vi "libssh2_session_hostkey.vi"(8 "error in (no error)":errorcluster, 11 "session":T1) -> (0 "error out":errorcluster, 1 "type":i32, 2 "hostkey":u8[](array[numeric]))   [LabVIEW 2017, in "libssh2.lvlib"]
doc: "Get the host key of the remote host.\n\nUse this output with libssh2_knownhost_checkp and continue only when the known host check result is MATCH."
uses:
  libssh2.lvlib
  Session Refnum.ctl
  Not A Session.vi
  <vilib>/Utility/error.llb/Error Cluster From Error Code.vi
  Global Settings.vi
  Read Session Refnum.vi
  <vilib>/Utility/semaphor.llb/Acquire Semaphore.vi
  <vilib>/Utility/semaphor.llb/Release Semaphore.vi
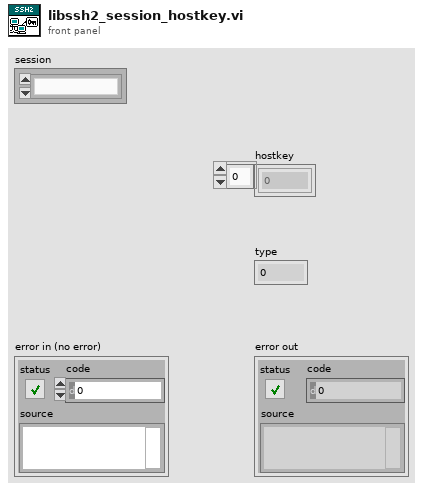
[diagram p1: front panel]
types:
  T1 = typedef "libssh2.lvlib/Session Refnum.ctl" = refnum<k1>
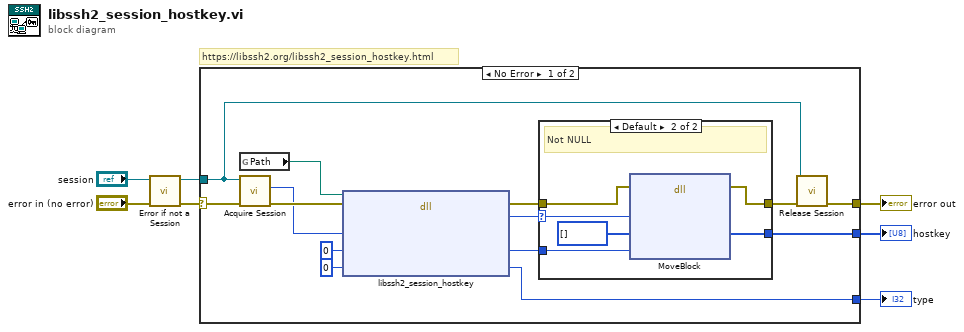
[diagram p0: block diagram]
diagram:
  # "https://libssh2.org/libssh2_session_hostkey.html"
  n1 = call "Error if not a Session.vi"("error in (no error)"="error in (no error)", "session"="session") -> ("error out"=w3:errorcluster, "session out"=w1:T1)  [unwired: 8 in]
  n2 = case shown="No Error" w3 {
    selector: w3 -> [w18 w29]
    tunnel: [w21 _] -> w7
    tunnel: [w9 w29] -> w6
    tunnel: [w19 _] -> w5
    tunnel: w1 -> [w8 _]
    frame No Error {
      n3 = global read "Global Settings.vi" "Path"() -> (w11:path)
      n4 = call "Acquire Session.vi"("error in (no error)"=w18, "session"=w8) -> ("error out"=w13:errorcluster, "LIBSSH2_SESSION*"=w12:u64)  [unwired: 7 in, 1 out]
      n5 = dll-call lib="?" fn="libssh2_session_hostkey"(path in=w11, error in=w13, "session"=w12, "len"=u64 0, "type"=0) -> (error out=w15:errorcluster, "return value"=w10:u64, "len"=w14:u64, "type"=w21:i32)  [unwired: 2 in, 1 out]
      n6 = case shown="Default" w10 {
        selector: w10 -> [_ w23]
        tunnel: w15 -> [w22 w28]
        tunnel: [w22 w27] -> w20
        tunnel: [_ w26] -> w19
        tunnel: w14 -> [_ w24]
        frame 0 {
          # "NULL"
        }
        frame Default {
          # "Not NULL"
          n7 = dll-call lib="LabVIEW" fn="MoveBlock"(error in=w28, "ps"=w23, "pd"=u8[] [], "size"=w24) -> (error out=w27:errorcluster, "pd"=w26:u8[])  [unwired: 5 in, 1 out]
        }
      }
      n8 = call "Release Session.vi"("error in (no error)"=w20, "session"=w8) -> ("error out"=w9:errorcluster)  [unwired: 9 in]
    }
    frame Error {
    }
  }
  "error out" <- w6
  "type" <- w7
  "hostkey" <- w5
